vi "csmdoc-Populate Example Description.vi"(8 "error in (no error)":errorcluster, 10 "Language Ring":string(combo)="English(EN)") -> (0 "error out":errorcluster)   [LabVIEW 2017, in "csmdoc.lvlib"]
uses:
  csmdoc.lvlib
  _Typedef/DocElement.ctl
  _Shared/CSM Shared.lvlib
  Communicable State Machine.lvlib
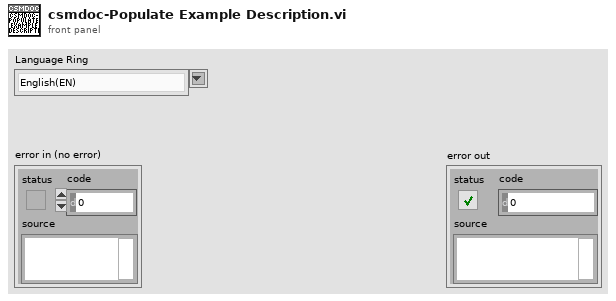
[diagram p1: front panel]
types:
  T1 = typedef "csmdoc.lvlib/DocNote.ctl" = cluster{"ID":string, "Content":string, "Type":string}
  T2 = typedef "csmdoc.lvlib/DocElement.ctl" = cluster{"ID":string, "Content":string[], "SubIDs":string[], "Path":string[]}
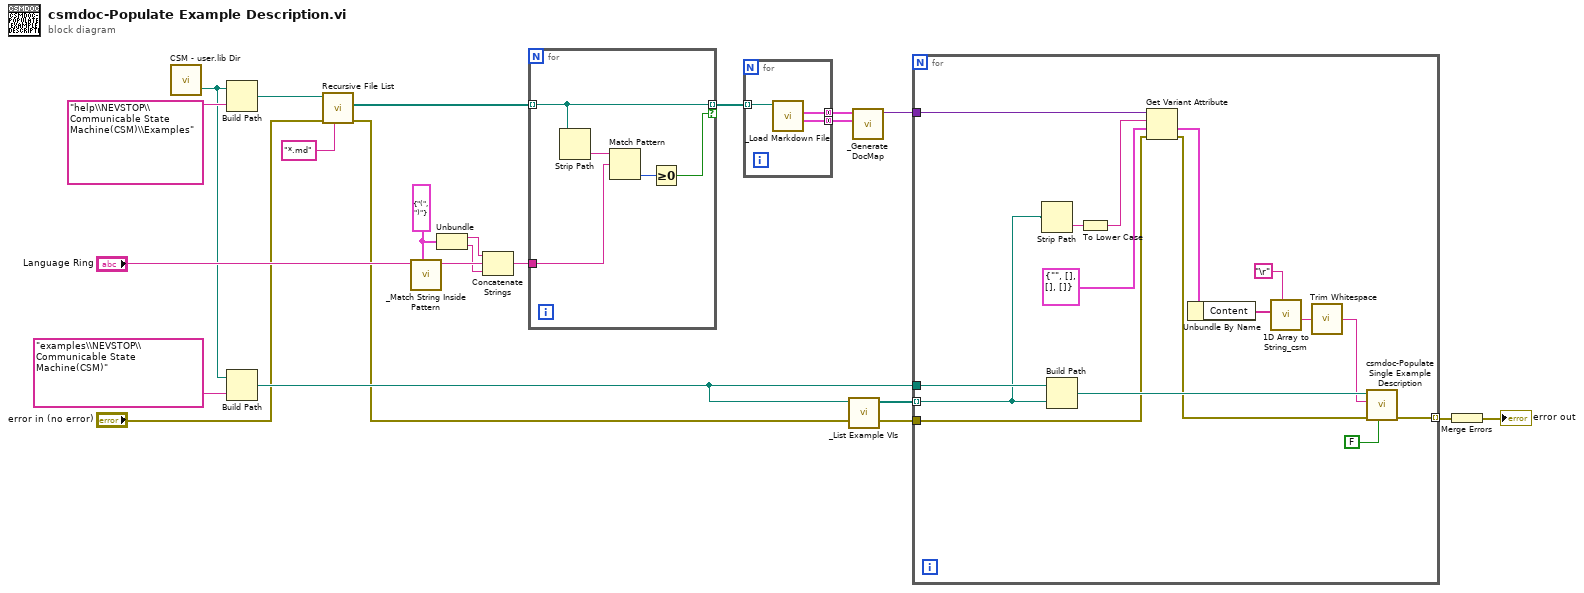
[diagram p0: block diagram]
diagram:
  w18 = cluster{"left":string, "right":string} {"left"="(", "right"=")"} ("Cluster")
  n1 = call "CSM - user.lib Dir.vi"() -> ("<LabVIEW>"=w3:path)  [unwired: 2 in, 1 out]
  n2 = Build Path(base path=w3, name or relative path="help\\NEVSTOP\\Communicable State Machine(CSM)\\Examples") -> (appended path=w21:path)
  n3 = Build Path(base path=w3, name or relative path="examples\\NEVSTOP\\Communicable State Machine(CSM)") -> (appended path=w8:path)
  n4 = call <vilib>:"Recursive File List.vi"("pattern"="*.md", "error in (no error)"="error in (no error)", "Folder Path"=w21) -> ("error out"=w5:errorcluster, "All Files in Dir"=w19:path[])  [unwired: 4 in, 3 out]
  n5 = call "_Match String Inside Pattern.vi"("Cluster"=w18, "string"="Language Ring") -> ("String inside"=w17:string)  [unwired: 9 in]
  n6 = Unbundle(w18) -> ("left"=w15:string, "right"=w16:string)
  n7 = Concatenate Strings(w15, w17, w16) -> (w14:string)
  n8 = for {
    tunnel: w19 -> [w27] mode=indexing
    tunnel: [w27] -> w10 mode=indexing if=w23
    tunnel: w14 -> [w25]
    n9 = Strip Path(path=w27) -> (name=w26:string)  [unwired: 1 out]
    n10 = Match Pattern(string=w26, regular expression=w25) -> (offset past match=w24:i32)  [unwired: 1 in, 3 out]
    n11 = Greater Or Equal To 0?(x=w24) -> (x >= 0?=w23:bool)
  }
  n12 = for {
    tunnel: w10 -> [w30] mode=indexing
    tunnel: [w29] -> w12 mode=concatenating
    tunnel: [w28] -> w11 mode=concatenating
    n13 = call "_Load Markdown File.vi"("Path"=w30) -> ("Array 2"=w28:T1[], "Array"=w29:T2[])  [unwired: 8 in, 1 out]
  }
  n14 = call "_List Example VIs.vi"("root"=w8) -> ("Array"=w6:path[])  [unwired: 10 in]
  n15 = call "_Generate DocMap.vi"("Array 2"=w11, "Array"=w12) -> ("Variant"=w7:variant)  [unwired: 9 in]
  n16 = for {
    tunnel: w8 -> [w36]
    tunnel: w7 -> [w35]
    tunnel: w6 -> [w34] mode=indexing
    tunnel: [w33] -> w2 mode=indexing
    tunnel: w5 -> [w31]
    n17 = Strip Path(path=w34) -> (name=w46:string)  [unwired: 1 out]
    n18 = Build Path(base path=w36, name or relative path=w34) -> (appended path=w40:path)
    n19 = To Lower Case(string=w46) -> (all lower case string=w45:string)
    n20 = Get Variant Attribute(Variant=w35, name=w45, default value (empty Variant)=T2 {"ID"="", "Content"=[], "SubIDs"=[], "Path"=[]} ("Cluster"), error in=w31) -> (value=w43:T2, error out=w32:errorcluster)  [unwired: 2 out]
    n21 = Unbundle By Name(w43) -> ("Content"=w42:string[])
    n22 = call "1D Array to String_csm.vi"("delimiter (Tab)"="\r", "Array of Strings"=w42) -> ("delimited string"=w38:string)  [unwired: 9 in]
    n23 = call <vilib>:"Trim Whitespace.vi"("string"=w38) -> ("trimmed string"=w37:string)  [unwired: 1 in]
    n24 = call "csmdoc-Populate Single Example Description.vi"("Show FP"=FALSE, "error in (no error)"=w32, "VI Description"=w37, "Path"=w40) -> ("error out"=w33:errorcluster)  [unwired: 7 in]
  }
  n25 = Merge Errors(w2) -> (→"error out":errorcluster)
